vi "StopICL.vi"(8 "error in (no error)":errorcluster, 11 "DeviceManager in":refnum<class "DeviceManager.lvclass">) -> (0 "error out":errorcluster, 3 "DeviceManager out":refnum<class "DeviceManager.lvclass">)   [LabVIEW 2023, in "DeviceManager.lvclass"]
uses:
  DeviceManager.lvclass
  DeviceManager.lvclass/DeviceManager.ctl
  88106aee-3f3d-4768-a856-6b02c0ac4dcc.vi
  <vilib>/JKI/JKI DotNet System Exec/dotnet_system_exec/dotnet_system_exec.lvclass
  Communicator/Communicator.lvclass
panel:
  # "Connector Pane"
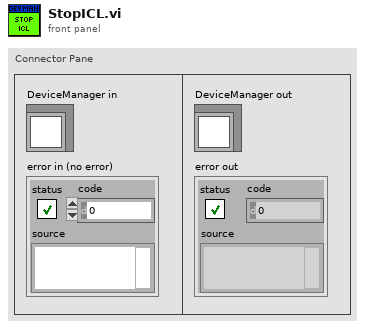
[diagram p1: front panel]
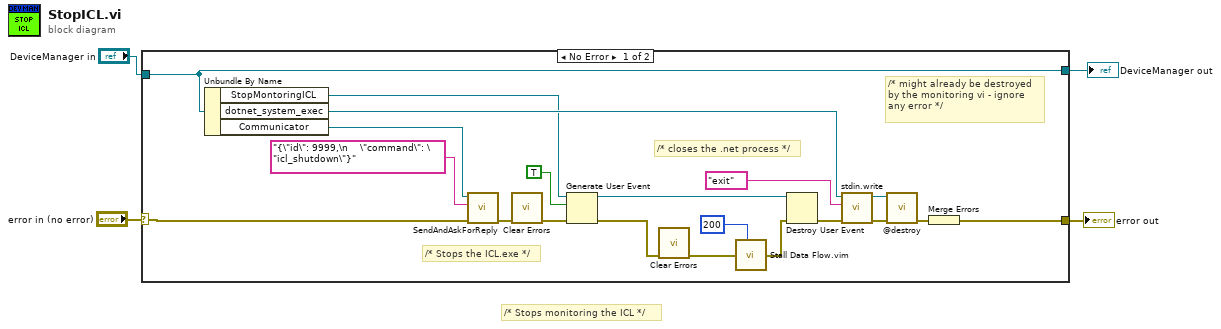
[diagram p0: block diagram]
diagram:
  # "/* Stops monitoring the ICL */"
  n1 = case shown="No Error" "error in (no error)" {
    selector: "error in (no error)" -> [w22 w26]
    tunnel: [w10 w26] -> w3
    tunnel: [w19 w25] -> w1
    tunnel: "DeviceManager in" -> [w19 w25]
    frame No Error {
      # "/* might already be destroyed\nby the monitoring vi - ignore \nany error */"
      # "/* closes the .net process */"
      # "/* Stops the ICL.exe */"
      n2 = Unbundle By Name(w19) -> ("StopMontoringICL"=w17:refnum<user-event>, "dotnet_system_exec"=w20:refnum<class "dotnet_system_exec.lvclass">, "Communicator"=w24:refnum<class "Communicator.lvclass">)
      n3 = call-dynamic "SendAndAskForReply.vi"("error in (no error)"=w22, "String to be sent"="{\"id\": 9999,\n    \"command\": \"icl_shutdown\"}", "Communicator in"=w24) -> ("error out"=w9:errorcluster)  [unwired: 6 in, 2 out]
      n4 = call <vilib>:"Clear Errors.vi"("error in (no error)"=w9) -> ("error out"=w7:errorcluster)  [unwired: 5 in, 1 out]
      n5 = Generate User Event(user event=w17, event data cluster=TRUE ("event data"), error in=w7) -> (user event out=w11:refnum<user-event>, error out=w15:errorcluster)  [unwired: 1 in]
      n6 = call <vilib>:"Clear Errors.vi"("error in (no error)"=w15) -> ("error out"=w14:errorcluster)  [unwired: 5 in, 1 out]
      n7 = call "Stall Data Flow.vim"("value in"=w14, "milliseconds to wait"=u32 200) -> ("value out"=w12:errorcluster)  [unwired: 1 out]
      n8 = Destroy User Event(user event=w11, error in=w12) -> (error out=w8:errorcluster)
      n9 = call-dynamic "stdin.write.vi"("error in (no error)"=w8, "stdin"="exit", "dotnet_system_exec in"=w20) -> ("error out"=w5:errorcluster, "dotnet_system_exec out"=w18:refnum<class "dotnet_system_exec.lvclass">)  [unwired: 7 in]
      n10 = call-dynamic "@destroy.vi"("error in (no error)"=w5, "dotnet_system_exec in"=w18) -> ("error out"=w6:errorcluster)  [unwired: 8 in, 1 out]
      n11 = Merge Errors(w6) -> (w10:errorcluster)
    }
    frame Error {
    }
  }
  "error out" <- w3
  "DeviceManager out" <- w1
